vi "CheckResultMatchResTest.vi"(8 "Your Suppose":i64[][](array[numeric]), 11 "Last Draw":i64[](array[numeric])) -> (0 "Matches":i32[](array[numeric]), 3 "Your Suppose":i64[][](array[numeric]))   [LabVIEW 2023]
panel:
  out "Last Draw":i64[](array[numeric])
  out "Result":i32[](array[numeric])
  out "Your Suppose":i32[][](array[numeric])
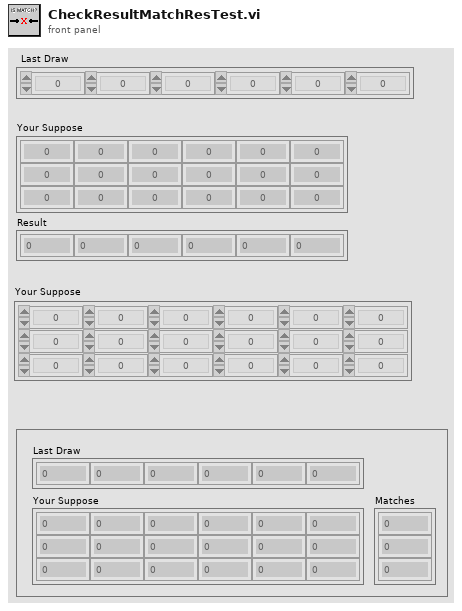
[diagram p1: front panel]
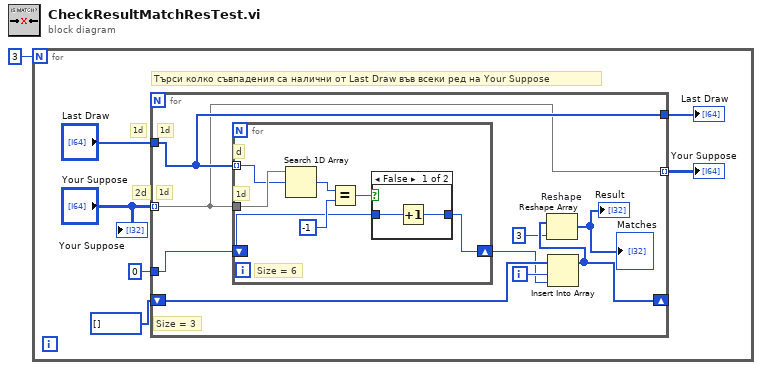
[diagram p0: block diagram]
diagram:
  n1 = for {
    N: 3 -> [_]
    # "Търси колко съвпадения са налични от Last Draw във всеки ред на Your Suppose"
    # "2d"
    # "1d"
    n2 = for {
      tunnel: "Your Suppose" -> [w11] mode=indexing
      tunnel: "Last Draw" -> [w12]
      shift-right: [w10] -> _
      shift-left: i32[] [] -> [w15]
      tunnel: 0 -> [w13]
      tunnel: [w12] -> w3
      tunnel: [w11] -> w2 mode=indexing
      i -> [w16]
      # "Size = 3"
      # "1d"
      # "1d"
      n3 = for {
        tunnel: w11 -> [w23]
        tunnel: w12 -> [w22] mode=indexing
        shift-right: [w18] -> w14
        shift-left: w13 -> [w17]
        # "Size = 6"
        # "1d"
        # "d"
        n4 = Search 1D Array(1D array=w23, element=w22) -> (index of element=w21:i32)  [unwired: 1 in]
        n5 = Equal?(x=w21, y=-1) -> (x = y?=w19:bool)
        n6 = case shown="False" w19 {
          tunnel: [w25 w26] -> w18
          tunnel: w17 -> [w24 w26]
          frame False {
            n7 = Increment(x=w24) -> (x+1=w25:i32)
          }
          frame True {
          }
        }
      }
      n8 = Insert Into Array "Insert Into Array"(array=w15, index=w16, new element=w14) -> (w10:i32[])
      n9 = Reshape Array "Reshape"(w10, 3 ("dimension size")) -> (→"Result" →"Matches":i32[])
    }
    "Last Draw" <- w3
    "Your Suppose" <- w2
    "Your Suppose" <- "Your Suppose"
  }
